vi "delete.vi"(4 "error in (no error)":errorcluster, 5 "timeout /ms (-1)":i32=-1, 6 "wait for activity? (F)":bool, 7 "objectRef":refnum<class "HGF_Reference.lvclass">) -> (0 "error out":errorcluster)   [LabVIEW 2012, in "HGF_ObjectManager.lvlib"]
doc: "Deinitialize and destroy an object and remove it from the global Object Manager database."
uses:
  HGF_ObjectManager.lvlib
  HGF_BaseClasses/HGF_Reference/HGF_Reference.lvclass
  HGF_BaseClasses/HGF_Factory/HGF_Factory.lvclass
  action.ctl
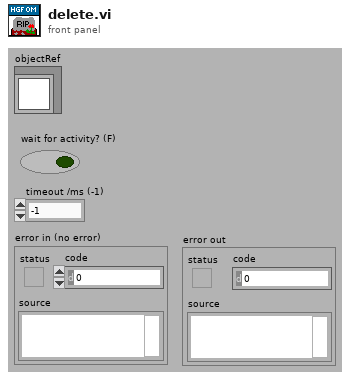
[diagram p1: front panel]
types:
  T1 = typedef "HGF_ObjectManager.lvlib/action.ctl" = enum16{"add", "remove", "name2ref", "ref2name ", "obj exists?", "cleanup", "get object list", "reset"}
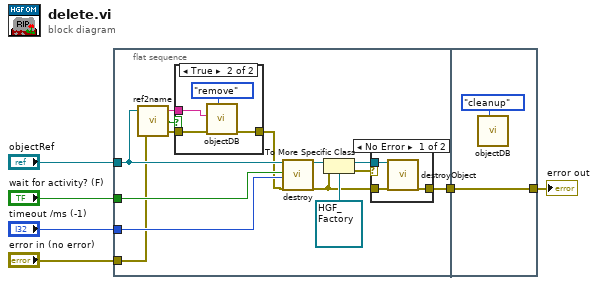
[diagram p0: block diagram]
diagram:
  n1 = flat-sequence {
    tunnel: "wait for activity? (F)" -> [w20]
    tunnel: "timeout /ms (-1)" -> [w19]
    tunnel: "error in (no error)" -> [w11]
    tunnel: "objectRef" -> [w12]
    tunnel: [w13] -> w1
    tunnel: w1 -> [w30]
    tunnel: [w30] -> w2
    frame #0 {
      n2 = call "ref2name.vi"("error in (no error)"=w11, "objectRef"=w12) -> ("error out"=w9:errorcluster, "obj exists"=w7:bool, "name out"=w10:string)  [unwired: 1 out]
      n3 = case shown="True" w7 {
        tunnel: w10 -> [_ w24]
        tunnel: w9 -> [w21 w23]
        tunnel: [w21 w22] -> w8
        frame False {
        }
        frame True {
          n4 = call "objectDB.vi"("Action"=action."remove", "error in (no error)"=w23, "name"=w24) -> ("error out"=w22:errorcluster)  [unwired: 2 in, 6 out]
        }
      }
      n5 = call "destroy.vi"("HGF_Reference"=w12, "wait for activity? (F)"=w20, "timeout /ms (-1)"=w19, "error in (no error)"=w8) -> ("Object"=w18:refnum<class>, "error out"=w14:errorcluster)  [unwired: 14 out]
      n6 = To More Specific Class(target class=refnum<class "HGF_Factory.lvclass"> refnum ("HGF_BaseClasses.lvlib:HGF_Factory.lvclass"), reference=w18, error in=w14) -> (specific class reference=w16:refnum<class "HGF_Factory.lvclass">, error out=w15:errorcluster)
      n7 = case shown="No Error" w15 {
        tunnel: w16 -> [w27 _]
        tunnel: w14 -> [w28 w29]
        tunnel: [w26 w29] -> w13
        frame No Error {
          n8 = call "destroyObject.vi"("HGF_Factory"=w27, "error in (no error)"=w28) -> ("error out"=w26:errorcluster)  [unwired: 17 out]
        }
        frame Error {
        }
      }
    }
    frame #1 {
      n9 = call "objectDB.vi"("Action"=action."cleanup") -> ()  [unwired: 4 in, 7 out]
    }
  }
  "error out" <- w2
